vi "SetCursorNamePosition XYGraph.vi"(1 "Graph":refnum<vi>) -> (0 "Graph Out":refnum<vi>)   [LabVIEW 2013, in "main.lvlib"]
uses:
  main.lvlib
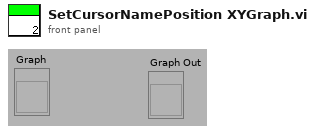
[diagram p1: front panel]
types:
  T1 = typedef "LVCursorListTypeDef.ctl" = cluster{"Name":string, "Color":u32, "Style":u8, "Point Style":u8, "Name Visible":bool, "Allow Drag":bool, "Cursor Mode":u32, "Plot":i32, "Index":i32, "Position":cluster{"X":dbl, "Y":dbl}, "X Scale":u32, "Y Scale":u32, "Watch Plots":i32[], "Watch All Plots":bool, "Plot Area":i32, "Label Offset":cluster{"X":dbl, "Y":dbl}}[]
  T2 = cluster{"Name":string, "Color":u32, "Style":u8, "Point Style":u8, "Name Visible":bool, "Allow Drag":bool, "Cursor Mode":u32, "Plot":i32, "Index":i32, "Position":cluster{"X":dbl, "Y":dbl}, "X Scale":u32, "Y Scale":u32, "Watch Plots":i32[], "Watch All Plots":bool, "Plot Area":i32, "Label Offset":cluster{"X":dbl, "Y":dbl}}
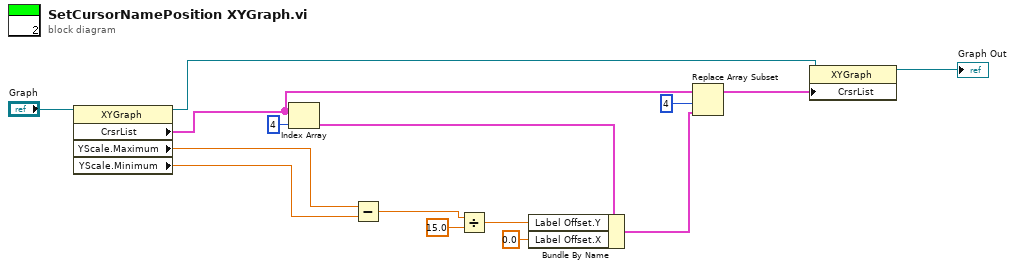
[diagram p0: block diagram]
diagram:
  n1 = property class="XYGraph"(reference="Graph") -> (reference out=w6:refnum<vi>, "CrsrList"=w9:T1, "YScale.Maximum"=w2:dbl, "YScale.Minimum"=w1:dbl)  [unwired: 1 in, 1 out]
  n2 = Index Array(array=w9, index=4) -> (element=w11:T2)
  n3 = Subtract(x=w2, y=w1) -> (x-y=w13:dbl)
  n4 = Divide(x=w13, y=15.0) -> (x/y=w10:dbl)
  n5 = Bundle By Name(cluster=w11, "Label Offset.Y"=w10, "Label Offset.X"=0.0) -> (w8:T2)
  n6 = Replace Array Subset(array=w9, new element=w8, index=4) -> (w5:T1)
  n7 = property class="XYGraph"(reference=w6, "CrsrList"=w5) -> (reference out=→"Graph Out":refnum<vi>)  [unwired: 1 in, 1 out]
